vi "setUp.vi"(8 "error in (no error)":errorcluster, 11 "reference in":refnum<class "Parameter Setting.lvclass">) -> (0 "error out":errorcluster, 3 "reference out":refnum<class "Parameter Setting.lvclass">)   [LabVIEW 2020, in "Static Errors Tests.lvlib" / "Parameter Setting.lvclass"]
doc: "setUp runs prior to the test method during test execution. Use this method to initialize any object data required by your tests."
uses:
  Parameter Setting.lvclass
  C:/Program Files (x86)/National Instruments/LabVIEW 2020/vi.lib/addons/_JKI Toolkits/VI Tester/TestCase.llb/TestCase.lvclass
  Parameter Setting.lvclass/Parameter Setting.ctl
  Source/VIs/New Error Cluster (256B).vi
  <vilib>/addons/_JKI Toolkits/VI Tester/TestCase.llb/TestCase.lvclass
  Source/Static Errors.lvlib
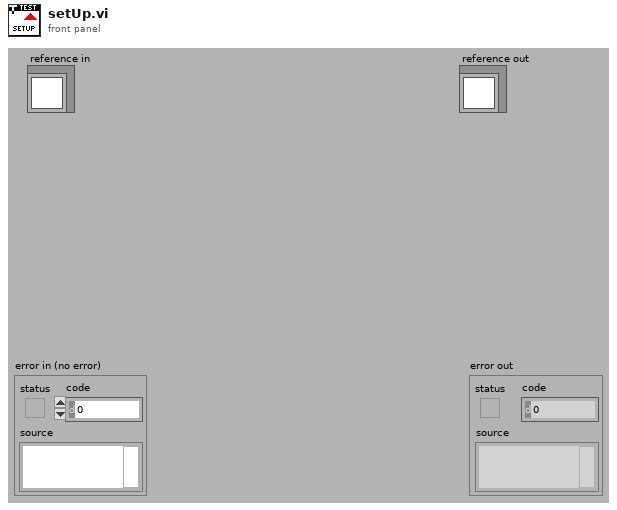
[diagram p1: front panel]
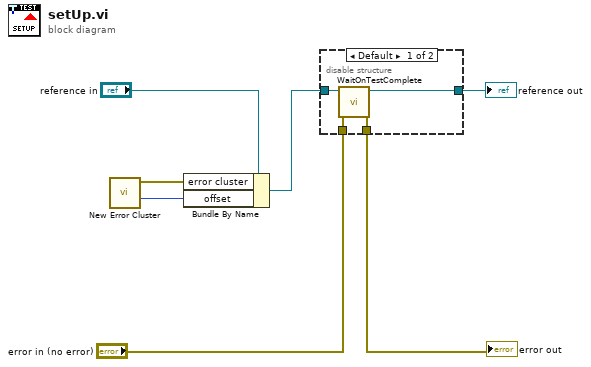
[diagram p0: block diagram]
diagram:
  n1 = call-poly "New Error Cluster.vi"() -> ("initial offset"=w1:i32, "error out"=w2:errorcluster)  [unwired: 10 in]
  n2 = Bundle By Name(cluster="reference in", "error cluster"=w2, "offset"=w1) -> (w3:refnum<class "Parameter Setting.lvclass">)
  n3 = disable-structure shown="Default" {
    disable-tunnel: "error in (no error)" -> [w11 w12]
    disable-tunnel: [w10 w12] -> w6
    disable-tunnel: [w9 w13] -> w4
    disable-tunnel: w3 -> [w8 w13]
    frame condition #0 (active) {
      n4 = call <vilib>:"WaitOnTestComplete.vi"("error in (no error)"=w11, "TestCase in"=w8) -> ("error out"=w10:errorcluster, "TestCase out"=w9:refnum<class "Parameter Setting.lvclass">)  [unwired: 8 in]
    }
    frame condition #1 {
    }
  }
  "error out" <- w6
  "reference out" <- w4
